vi "Frame Process.vi"(8 "error in (no error)":errorcluster, 10 "Video Frame In":refnum<class "Video Frame.lvclass">, 11 "Video Processor in":refnum<class "Video Cam Processor.lvclass">) -> (0 "error out":errorcluster, 3 "Video Processor out":refnum<class "Video Cam Processor.lvclass">)   [LabVIEW 2018, in "Video Cam Processor.lvclass"]
uses:
  Video Cam Processor.lvclass
  Video Frame/Video Frame.lvclass
  Video Cam Processor.lvclass/Video Cam Processor.ctl
  2c118313-fc59-40f1-b07d-4322096fb157.vi
  5fbe6361-8a29-4a31-af02-72406432bcc9.vi
  6936c895-b0a3-4e2c-9892-7cf1b7938e16.vi
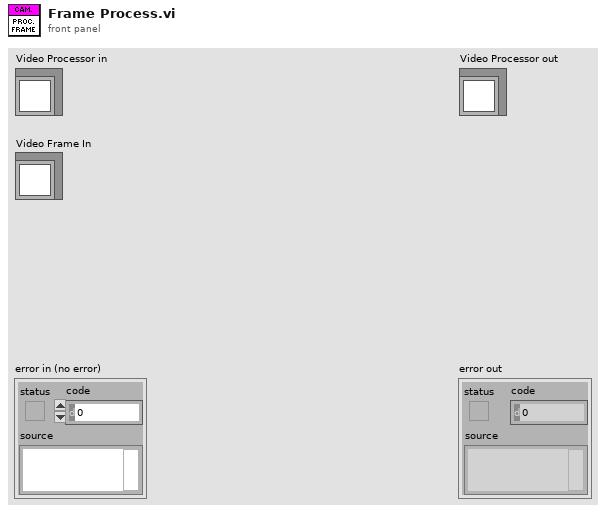
[diagram p1: front panel]
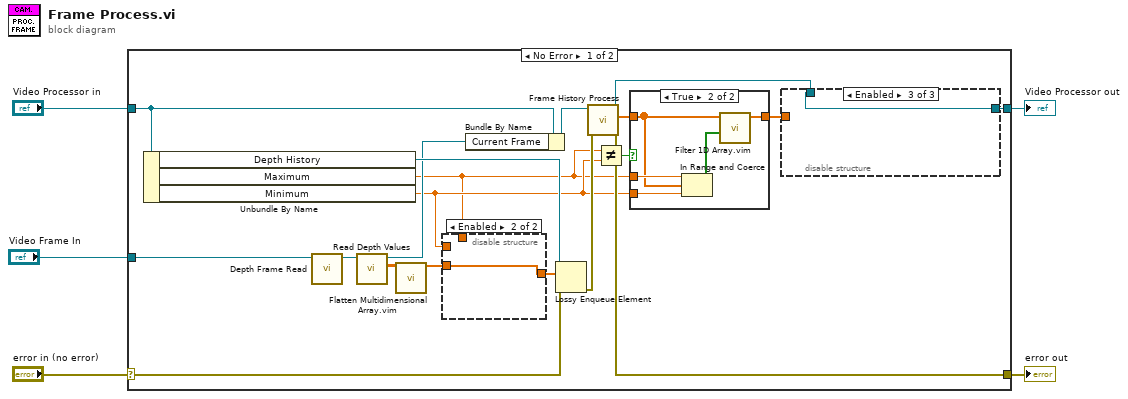
[diagram p0: block diagram]
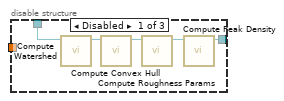
[diagram p2: hidden frame]
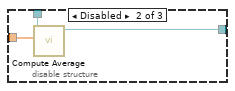
[diagram p3: hidden frame]
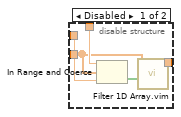
[diagram p5: hidden frame]
diagram:
  n1 = case shown="No Error" "error in (no error)" {
    selector: "error in (no error)" -> [w17 w47]
    tunnel: [w15 w47] -> w4
    tunnel: [w6 w46] -> w2
    tunnel: "Video Processor in" -> [w19 w46]
    tunnel: "Video Frame In" -> [w18 _]
    frame No Error {
      n2 = Unbundle By Name(w19) -> ("Depth History"=w24:refnum<queue>, "Maximum"=w7:dbl, "Minimum"=w8:dbl)
      n3 = call-dynamic "Depth Frame Read.vi"("Video Frame in"=w18) -> ("Video Frame out"=w14:refnum<class "Video Frame.lvclass">)  [unwired: 6 in, 4 out]
      n4 = call-dynamic "Read Depth Values.vi"("Video Frame in"=w14) -> ("Depth Values"=w12:dbl[][], "Video Frame out"=w13:refnum<class "Video Frame.lvclass">)  [unwired: 8 in, 1 out]
      n5 = call "Flatten Multidimensional Array.vim"("Array"=w12) -> ("output array"=w11:dbl[])  [unwired: 14 in]
      n6 = disable-structure shown="Enabled" {
        disable-tunnel: w7 -> [w44 _]
        disable-tunnel: w8 -> [w43 _]
        disable-tunnel: w11 -> [w42 w45]
        disable-tunnel: [w40 w45] -> w20
        frame Disabled {
          n7 = In Range and Coerce(upper limit=w44, x=w42, lower limit=w43) -> (In Range?=w41:bool[])  [unwired: 1 out]
          n8 = call "Filter 1D Array.vim"("Boolean Filter"=w41, "Array"=w42) -> ("Array Out"=w40:dbl[])  [unwired: 9 in]
        }
        frame Enabled {
        }
      }
      n9 = Bundle By Name(cluster=w19, "Current Frame"=w13) -> (w23:refnum<class "Video Cam Processor.lvclass">)
      n10 = Lossy Enqueue Element(queue=w24, element=w20, error in (no error)=w17) -> (error out=w16:errorcluster)  [unwired: 3 out]
      n11 = call-dynamic "Frame History Process.vi"("error in (no error)"=w16, "Video Processor in"=w23) -> ("error out"=w15:errorcluster, "Depth Values Out"=w10:dbl[], "Video Processor out"=w22:refnum<class "Video Cam Processor.lvclass">)  [unwired: 7 in]
      n12 = Not Equal?(x=w7, y=w8) -> (x != y?=w9:bool)
      n13 = case shown="True" w9 {
        tunnel: [w34 w36] -> w21
        tunnel: w10 -> [w34 w35]
        tunnel: w7 -> [_ w38]
        tunnel: w8 -> [_ w37]
        frame False {
        }
        frame True {
          n14 = In Range and Coerce(upper limit=w38, x=w35, lower limit=w37) -> (In Range?=w39:bool[])  [unwired: 1 out]
          n15 = call "Filter 1D Array.vim"("Boolean Filter"=w39, "Array"=w35) -> ("Array Out"=w36:dbl[])  [unwired: 9 in]
        }
      }
      n16 = disable-structure shown="Enabled" {
        disable-tunnel: w22 -> [w29 w32 w33]
        disable-tunnel: w21 -> [_ w31 _]
        disable-tunnel: [w27 w30 w33] -> w6
        frame Disabled {
          n17 = call-dynamic "Compute Watershed.vi"("Video Cam Processor in"=w29) -> ("Video Cam Processor out"=w26:refnum<class "Video Cam Processor.lvclass">)  [unwired: 8 in, 2 out]
          n18 = call-dynamic "Compute Convex Hull.vi"("Video Cam Processor in"=w26) -> ("Video Cam Processor out"=w25:refnum<class "Video Cam Processor.lvclass">)  [unwired: 9 in, 1 out]
          n19 = call-dynamic "Compute Roughness Params.vi"("Video Cam Processor in"=w25) -> ("Video Cam Processor out"=w28:refnum<class "Video Cam Processor.lvclass">)  [unwired: 9 in, 1 out]
          n20 = call-dynamic "Compute Peak Density.vi"("Video Cam Processor in"=w28) -> ("Video Cam Processor out"=w27:refnum<class "Video Cam Processor.lvclass">)  [unwired: 8 in, 2 out]
        }
        frame Disabled {
          n21 = call-dynamic "Compute Average.vi"("Data"=w31, "Video Processor in"=w32) -> ("Video Processor out"=w30:refnum<class "Video Cam Processor.lvclass">)  [unwired: 8 in, 1 out]
        }
        frame Enabled {
        }
      }
    }
    frame Error {
    }
  }
  "error out" <- w4
  "Video Processor out" <- w2
